vi "Datalog to ASCII (STATE_).vi"(4 "Error in":errorcluster, 5 "ASCII output path":path=path "C:/Datalogs/Log1_S_.txt", 6 "Precision":i16=4, 7 "Datalog path":path=path "C:/Datalogs/Log1_S_.log") -> (0 "Error out":errorcluster)   [LabVIEW 2015]
uses:
  Ctls/All state values (for datalog).ctl
  Ctls/Environmental state values.ctl
  Ctls/Inertial state values.ctl
  <vilib>/Utility/file.llb/Write Delimited Spreadsheet (string).vi
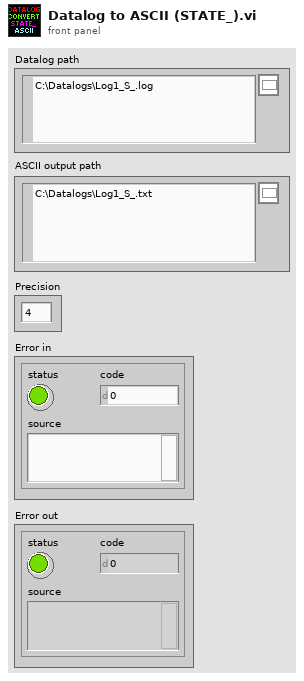
[diagram p1: front panel]
types:
  T1 = typedef "All state values (for datalog).ctl" = cluster{"Time Stamp":timestamp, "dt (ms)":i32, "Environmental state values":T2, "Inertial state values":T3}
  T2 = typedef "Environmental state values.ctl" = cluster{"Thermistor (degC)":sgl, "Sensor temp. (degC)":sgl, "P_atmos (Pa)":sgl, "Rel. Humidity (%)":sgl, "Density (kg/m^3)":sgl, "Dew point (degC)":sgl, "Pressure alt. (m)":sgl, "Density alt. (m)":sgl}
  T3 = typedef "Inertial state values.ctl" = cluster{"w_x (dps)":sgl, "w_y (dps)":sgl, "w_z (dps)":sgl, "a_x (g)":sgl, "a_y (g)":sgl, "a_z (g)":sgl, "Stale sample":u8, "Sensor temp. (degC)":sgl}
  T4 = enum16{"open", "replace", "create", "open or create", "replace or create", "replace or create with confirmation"}
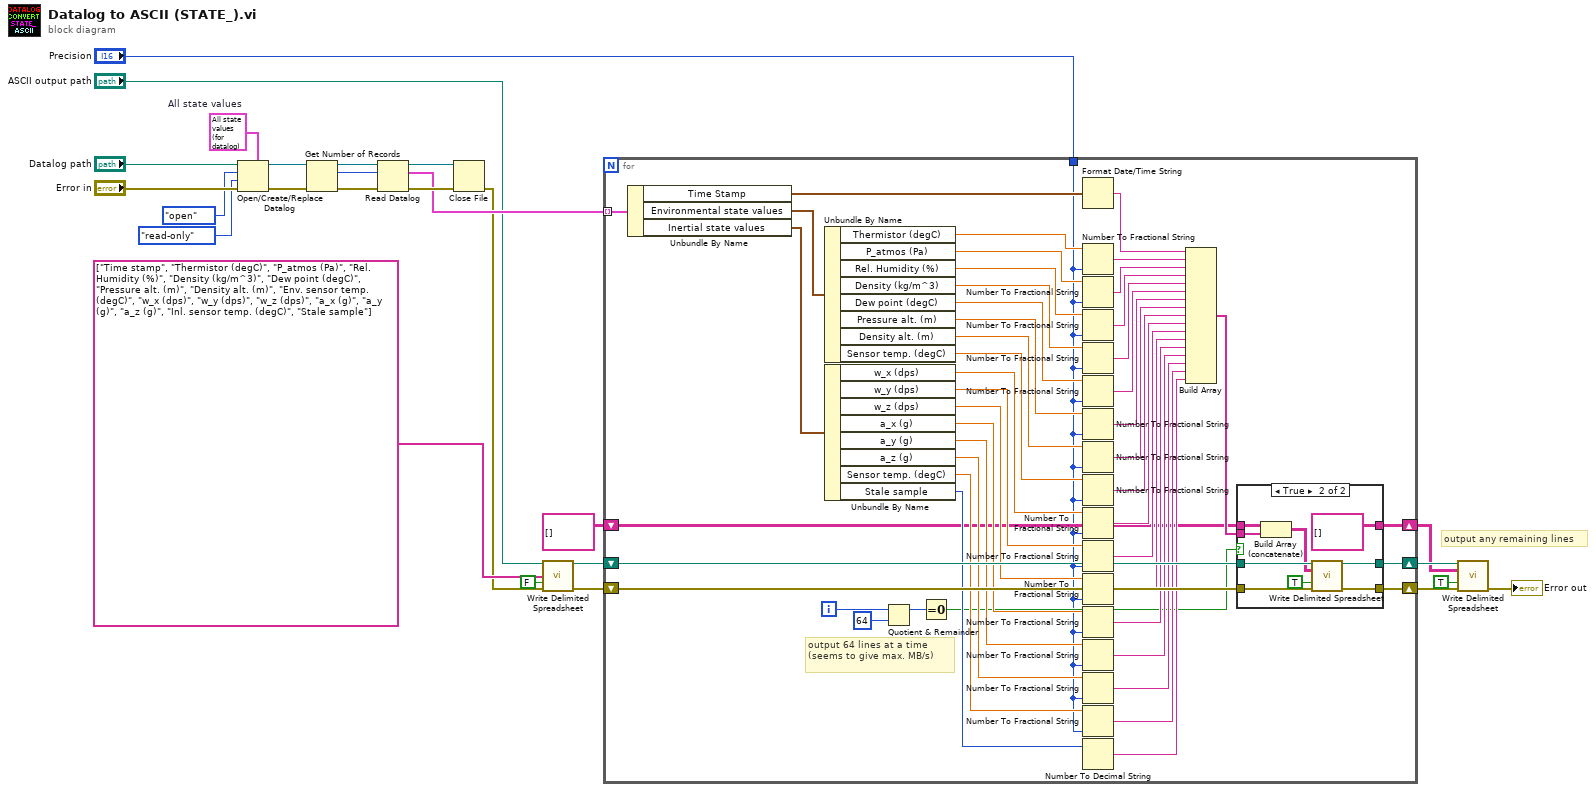
[diagram p0: block diagram]
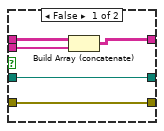
[diagram p2: hidden frame]
diagram:
  w13 = T1 {"Time Stamp"=timestamp(0 s since 1904-01-01), "dt (ms)"=0, "Environmental state values"={"Thermistor (degC)"=0.0, "Sensor temp. (degC)"=0.0, "P_atmos (Pa)"=0.0, "Rel. Humidity (%)"=0.0, "Density (kg/m^3)"=0.0, "Dew point (degC)"=0.0, "Pressure alt. (m)"=0.0, "Density alt. (m)"=0.0}, "Inertial state values"={"w_x (dps)"=0.0, "w_y (dps)"=0.0, "w_z (dps)"=0.0, "a_x (g)"=0.0, "a_y (g)"=0.0, "a_z (g)"=0.0, "Stale sample"=0, "Sensor temp. (degC)"=0.0}}  # All state values
  # "output any remaining lines"
  n1 = Open/Create/Replace Datalog(5:w13, 8:"Error in", 9:enum16{"read/write", "read-only", "write-only"}."read-only" ("access (0:read/write)"), 10:T4."open" ("operation (0:open)"), 11:"Datalog path") -> (0:w21:errorcluster, 3:w22:refnum<k1>)  [unwired: 1 in, 1 out]
  n2 = Get Number of Records(4:w21, 7:w22) -> (0:w18:errorcluster, 2:w19:i64, 3:w20:refnum<k1>)
  n3 = Read Datalog(4:w18, 6:w19, 7:w20) -> (0:w16:errorcluster, 2:w15:T1[], 3:w17:refnum<k1>)
  n4 = Close File(refnum=w17, error in=w16) -> (error out=w9:errorcluster)  [unwired: 1 out]
  n5 = call-poly <vilib>:"Write Delimited Spreadsheet.vi"("file path (dialog if empty)"="ASCII output path", "1D data"=string[] ["Time stamp", "Thermistor (degC)", "P_atmos (Pa)", "Rel. Humidity (%)", "Density (kg/m^3)", "Dew point (degC)", "Pressure alt. (m)", "Density alt. (m)", "Env. sensor temp. (degC)", "w_x (dps)", "w_y (dps)", "w_z (dps)", "a_x (g)", "a_y (g)", "a_z (g)", "Inl. sensor temp. (degC)", "Stale sample"], "append to file? (F)"=FALSE, "error in (no error)"=w9) -> ("new file path (Not A Path if cancelled)"=w7:path, "error out"=w6:errorcluster)  [unwired: 10 in]
  n6 = for {
    tunnel: w15 -> [w58] mode=indexing
    tunnel: "Precision" -> [w27]
    shift-right: [w33] -> w5
    shift-left: w7 -> [w74]
    shift-right: [w32] -> w4
    shift-left: w6 -> [w75]
    shift-right: [w30] -> w1
    shift-left: string[][] [] -> [w29]
    i -> [w34]
    # "output 64 lines at a time (seems to give max. MB/s)"
    n7 = Unbundle By Name(w58) -> ("Time Stamp"=w57:timestamp, "Environmental state values"=w56:T2, "Inertial state values"=w55:T3)
    n8 = Unbundle By Name(w56) -> ("Thermistor (degC)"=w54:sgl, "P_atmos (Pa)"=w53:sgl, "Rel. Humidity (%)"=w52:sgl, "Density (kg/m^3)"=w51:sgl, "Dew point (degC)"=w50:sgl, "Pressure alt. (m)"=w49:sgl, "Density alt. (m)"=w48:sgl, "Sensor temp. (degC)"=w47:sgl)
    n9 = Unbundle By Name(w55) -> ("w_x (dps)"=w46:sgl, "w_y (dps)"=w45:sgl, "w_z (dps)"=w44:sgl, "a_x (g)"=w43:sgl, "a_y (g)"=w42:sgl, "a_z (g)"=w41:sgl, "Sensor temp. (degC)"=w40:sgl, "Stale sample"=w39:u8)
    n10 = Quotient & Remainder(x=w34, y=64) -> (x-y*floor(x/y)=w36:i32)  [unwired: 1 out]
    n11 = Equal To 0?(x=w36) -> (x = 0?=w28:bool)
    n12 = Format Date/Time String(seconds (now)=w57) -> (date/time string=w66:string)  [unwired: 2 in]
    n13 = Number To Fractional String(number=w54, precision (6)=w27) -> (F-format string=w73:string)  [unwired: 2 in]
    n14 = Number To Fractional String(number=w53, precision (6)=w27) -> (F-format string=w72:string)  [unwired: 2 in]
    n15 = Number To Fractional String(number=w52, precision (6)=w27) -> (F-format string=w71:string)  [unwired: 2 in]
    n16 = Number To Fractional String(number=w51, precision (6)=w27) -> (F-format string=w70:string)  [unwired: 2 in]
    n17 = Number To Fractional String(number=w50, precision (6)=w27) -> (F-format string=w69:string)  [unwired: 2 in]
    n18 = Number To Fractional String(number=w49, precision (6)=w27) -> (F-format string=w68:string)  [unwired: 2 in]
    n19 = Number To Fractional String(number=w48, precision (6)=w27) -> (F-format string=w67:string)  [unwired: 2 in]
    n20 = Number To Fractional String(number=w47, precision (6)=w27) -> (F-format string=w65:string)  [unwired: 2 in]
    n21 = Number To Fractional String(number=w46, precision (6)=w27) -> (F-format string=w64:string)  [unwired: 2 in]
    n22 = Number To Fractional String(number=w45, precision (6)=w27) -> (F-format string=w63:string)  [unwired: 2 in]
    n23 = Number To Fractional String(number=w44, precision (6)=w27) -> (F-format string=w62:string)  [unwired: 2 in]
    n24 = Number To Fractional String(number=w43, precision (6)=w27) -> (F-format string=w61:string)  [unwired: 2 in]
    n25 = Number To Fractional String(number=w42, precision (6)=w27) -> (F-format string=w60:string)  [unwired: 2 in]
    n26 = Number To Fractional String(number=w41, precision (6)=w27) -> (F-format string=w59:string)  [unwired: 2 in]
    n27 = Number To Fractional String(number=w40, precision (6)=w27) -> (F-format string=w38:string)  [unwired: 2 in]
    n28 = Number To Decimal String(number=w39) -> (decimal integer string=w37:string)  [unwired: 1 in]
    n29 = Build Array(w66, w73, w72, w71, w70, w69, w68, w67, w65, w64, w63, w62, w61, w60, w59, w38, w37) -> (w31:string[])
    n30 = case shown="True" w28 {
      tunnel: [w78 string[][] []] -> w30
      tunnel: [w77 w88] -> w33
      tunnel: [w76 w87] -> w32
      tunnel: w74 -> [w77 w85]
      tunnel: w75 -> [w76 w84]
      tunnel: w31 -> [w79 w83]
      tunnel: w29 -> [w80 w82]
      frame False {
        n31 = Build Array (concatenate)(w80, w79) -> (w78:string[][])
      }
      frame True {
        n32 = Build Array (concatenate)(w82, w83) -> (w81:string[][])
        n33 = call-poly <vilib>:"Write Delimited Spreadsheet.vi"("file path (dialog if empty)"=w85, "2D data"=w81, "append to file? (F)"=TRUE, "error in (no error)"=w84) -> ("new file path (Not A Path if cancelled)"=w88:path, "error out"=w87:errorcluster)  [unwired: 10 in]
      }
    }
  }
  n34 = call-poly <vilib>:"Write Delimited Spreadsheet.vi"("file path (dialog if empty)"=w5, "2D data"=w1, "append to file? (F)"=TRUE, "error in (no error)"=w4) -> ("error out"=→"Error out":errorcluster)  [unwired: 10 in, 1 out]
